vi "data beautifier.vi"(6 "Y-wave columns":u8[](array[numeric])=[4], 7 "X-wave column":u8, 8 "data cluster":cluster{"all rows":dbl[][]}[](array[cluster])=[{"all rows"=array3962x7[27734 elements]}, {"all rows"=array19075x7[133525 elements]}, {"all rows"=array4476x7[31332 elements]}], 9 "show files":T2(array[cluster])=[{"String"="sa_cryst,,_2nd.001", "Boolean"=TRUE, "begin"=0, "length"=3962, "y weight"=1.0}, {"String"="sa_cryst,,_2nd.002", "Boolean"=FALSE, "begin"=0, "length"=19075, "y weight"=1.0}, {"String"="sa_cryst,,_2nd.003", "Boolean"=TRUE, "begin"=0, "length"=4476, "y weight"=1.0}]) -> (0 "result data cluster":cluster{"all rows":dbl[][]}[](array[cluster]))   [LabVIEW 2019]
panel:
  in  "remove bad data pts":bool
  in  "remove duplicates":bool
  in  "cancel":bool
  in  "remove zero":bool
  out "XY Graph 2":T1(graph)
  in  "OK Button":bool
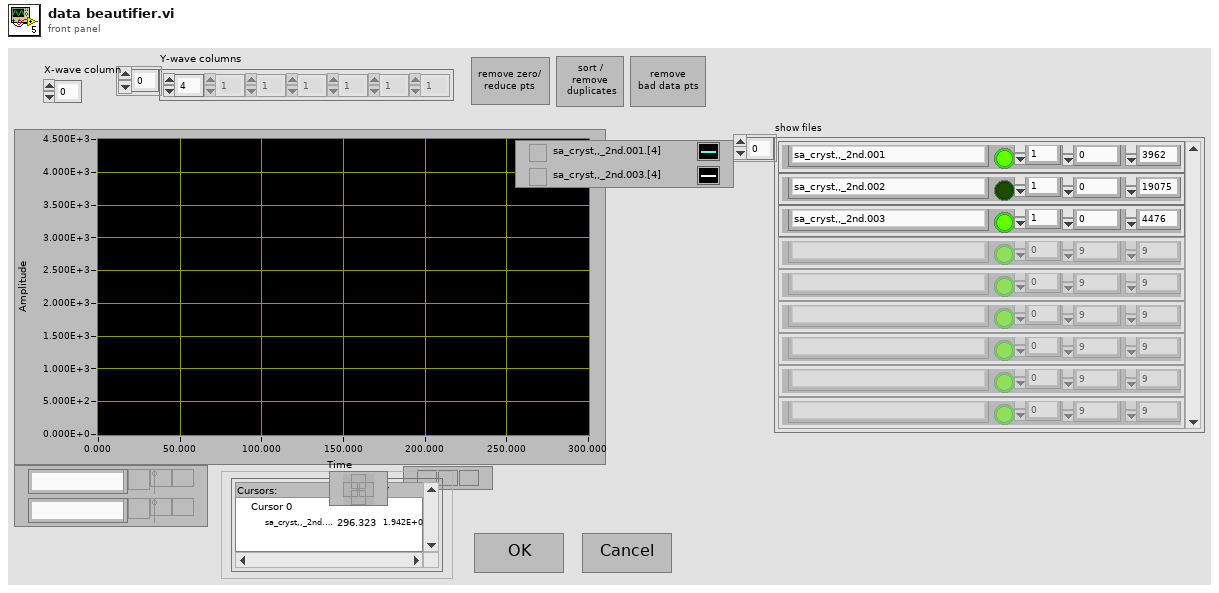
[diagram p1: front panel]
types:
  T1 = cluster{"indep array (x) out":dbl[], "dep array (y) out":dbl[]}[]
  T2 = cluster{"String":string, "Boolean":bool, "begin":u32, "length":u32, "y weight":dbl}[]
  T3 = cluster{"show files":cluster{"String":string, "Boolean":bool, "begin":u32, "length":u32, "y weight":dbl}[], "data cluster":cluster{"all rows":dbl[][]}[], "new dataset?":bool}
  T4 = cluster{"String":string, "Boolean":bool, "begin":u32, "end":u32, "Numeric":dbl}[]
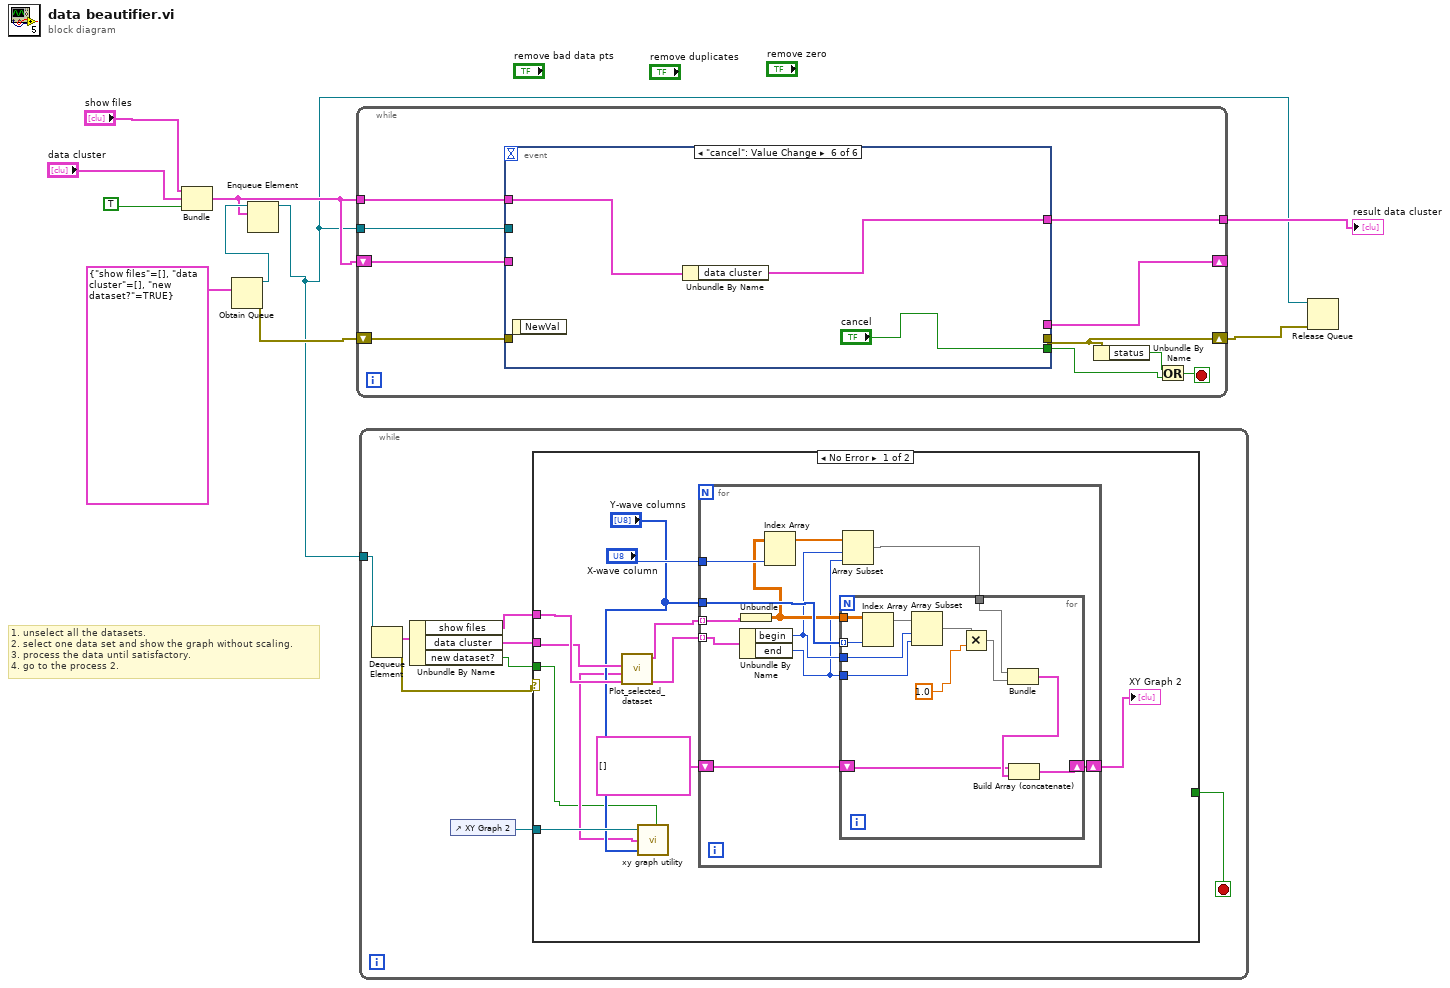
[diagram p0: block diagram]
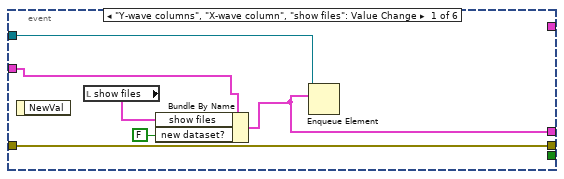
[diagram p2: hidden frame]
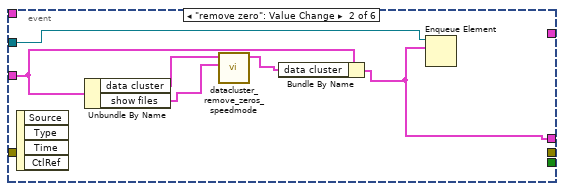
[diagram p3: hidden frame]
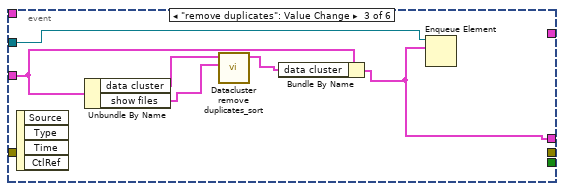
[diagram p4: hidden frame]
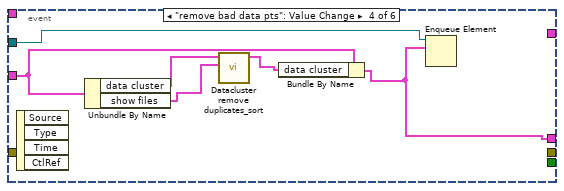
[diagram p5: hidden frame]
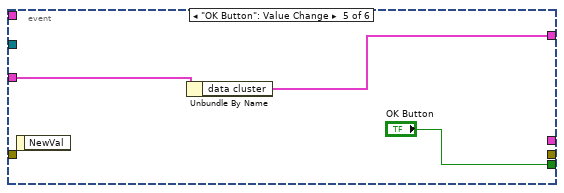
[diagram p6: hidden frame]
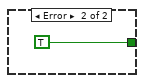
[diagram p7: hidden frame]
diagram:
  # "1. unselect all the datasets.\n2. select one data set and show the graph without scaling.\n3. process the data until satisfactory.\n4. go to the process 2."
  n1 = Bundle("show files"="show files", "data cluster"="data cluster", "new dataset?"=TRUE) -> (w3:T3)  [unwired: 1 in]
  n2 = Obtain Queue(element data type=T3 {"show files"=[], "data cluster"=[], "new dataset?"=TRUE}) -> (queue out=w4:refnum<queue>, error out=w9:errorcluster)  [unwired: 4 in, 1 out]
  n3 = Enqueue Element(queue=w4, element=w3) -> (queue out=w2:refnum<queue>)  [unwired: 2 in, 2 out]
  n4 = while {
    tunnel: w2 -> [w20]
    shift-right: [w19] -> _
    shift-left: w3 -> [w14]
    shift-right: [w13] -> w6
    shift-left: w9 -> [w18]
    tunnel: [w12] -> w5
    tunnel: w3 -> [w11]
    stop <- w15 stop-if-true
    n5 = event shown="[5] \"cancel\": Value Change" {
      selector: _ -> [_ _ _ _ _ _]
      dyn-events: _ -> [_ _ _ _ _ _]
      timeout: _ -> [_ _ _ _ _ _]
      tunnel: w20 -> [w26 w28 w34 w40 _ _]
      tunnel: [w23 w27 w33 w39 _ _] -> w19
      tunnel: w18 -> [w25 _ _ _ _ _]
      tunnel: [w25 _ _ _ _ _] -> w13
      tunnel: [_ _ _ _ "OK Button" "cancel"] -> w16
      tunnel: w14 -> [w22 w30 w36 w42 w46 _]
      tunnel: [_ _ _ _ w45 w50] -> w12
      tunnel: w11 -> [_ _ _ _ _ w48]
      event "Y-wave columns", "X-wave column", "show files": Value Change {
        n6 = event-data() -> ()  [unwired: 1 in, 1 out]
        n7 = local read "show files"() -> (w24:T2)
        n8 = Bundle By Name(cluster=w22, "show files"=w24, "new dataset?"=FALSE) -> (w23:T3)
        n9 = Enqueue Element(queue=w26, element=w23) -> ()  [unwired: 2 in, 3 out]
      }
      event "remove zero": Value Change {
        n10 = event-data() -> ()  [unwired: 1 in, 4 out]
        n11 = Unbundle By Name(w30) -> ("data cluster"=w31:cluster{"all rows":dbl[][]}[], "show files"=w32:T2)
        n12 = call "datacluster_remove_zeros_speedmode.vi"("Datasets to be processed"=w32, "data cluster"=w31) -> ("data cluster out"=w29:cluster{"all rows":dbl[][]}[])  [unwired: 9 in]
        n13 = Bundle By Name(cluster=w30, "data cluster"=w29) -> (w27:T3)
        n14 = Enqueue Element(queue=w28, element=w27) -> ()  [unwired: 2 in, 3 out]
      }
      event "remove duplicates": Value Change {
        n15 = event-data() -> ()  [unwired: 1 in, 4 out]
        n16 = Unbundle By Name(w36) -> ("data cluster"=w37:cluster{"all rows":dbl[][]}[], "show files"=w38:T2)
        n17 = call "Datacluster remove duplicates_sort.vi"("Datasets to be processed"=w38, "data cluster"=w37) -> ("data cluster out"=w35:cluster{"all rows":dbl[][]}[])  [unwired: 9 in]
        n18 = Bundle By Name(cluster=w36, "data cluster"=w35) -> (w33:T3)
        n19 = Enqueue Element(queue=w34, element=w33) -> ()  [unwired: 2 in, 3 out]
      }
      event "remove bad data pts": Value Change {
        n20 = event-data() -> ()  [unwired: 1 in, 4 out]
        n21 = Unbundle By Name(w42) -> ("data cluster"=w43:cluster{"all rows":dbl[][]}[], "show files"=w44:T2)
        n22 = call "Datacluster remove duplicates_sort.vi"("Datasets to be processed"=w44, "data cluster"=w43) -> ("data cluster out"=w41:cluster{"all rows":dbl[][]}[])  [unwired: 9 in]
        n23 = Bundle By Name(cluster=w42, "data cluster"=w41) -> (w39:T3)
        n24 = Enqueue Element(queue=w40, element=w39) -> ()  [unwired: 2 in, 3 out]
      }
      event "OK Button": Value Change {
        n25 = event-data() -> ()  [unwired: 1 in, 1 out]
        n26 = Unbundle By Name(w46) -> ("data cluster"=w45:cluster{"all rows":dbl[][]}[])
      }
      event "cancel": Value Change {
        n27 = event-data() -> ()  [unwired: 1 in, 1 out]
        n28 = Unbundle By Name(w48) -> ("data cluster"=w50:cluster{"all rows":dbl[][]}[])
      }
    }
    n29 = Unbundle By Name(w13) -> ("status"=w17:bool)
    n30 = Or(x=w17, y=w16) -> (x .or. y?=w15:bool)
  }
  "result data cluster" <- w5
  n31 = while {
    tunnel: w2 -> [w58]
    stop <- w53 stop-if-true
    n32 = Dequeue Element(queue=w58) -> (element=w57:T3, error out=w54:errorcluster)  [unwired: 2 in, 2 out]
    n33 = Unbundle By Name(w57) -> ("show files"=w55:T2, "data cluster"=w56:cluster{"all rows":dbl[][]}[], "new dataset?"=w51:bool)
    n34 = control-ref of="XY Graph 2"() -> (w52:refnum<vi>)
    n35 = case shown="No Error" w54 {
      tunnel: w56 -> [w64 _]
      tunnel: w55 -> [w65 _]
      tunnel: [_ TRUE] -> w53
      tunnel: w52 -> [w62 _]
      tunnel: w51 -> [w59 _]
      frame No Error {
        n36 = call "Plot_selected_dataset.vi"("input xy data arrays"=w64, "file names and switch"=w65) -> ("show files out"=w60:T4, "selected xy data arrays"=w63:cluster{"all rows":dbl[][]}[], "selected showfiles"=w66:T4)  [unwired: 1 in, 4 out]
        n37 = call "xy graph utility.vi"("redraw?"=w59, "y-wave columns"="Y-wave columns", "show files"=w60, "XYGraph Refnum"=w62) -> ()  [unwired: 1 in]
        n38 = for {
          tunnel: "Y-wave columns" -> [w80]
          tunnel: "X-wave column" -> [w79]
          tunnel: w63 -> [w72] mode=indexing
          tunnel: w66 -> [w71] mode=indexing
          shift-right: [w73] -> w68
          shift-left: cluster{dbl[], dbl[]}[] [] -> [w70]
          n39 = Unbundle By Name(w71) -> ("begin"=w76:u32, "end"=w75:u32)
          n40 = Unbundle(w72) -> ("all rows"=w78:dbl[][])
          n41 = Index Array(array=w78, index (col)=w79) -> (element=w77:dbl[])  [unwired: 1 in]
          n42 = Array Subset(array=w77, index=w76, length=w75) -> (w74:dbl[])
          n43 = for {
            tunnel: w78 -> [w92]
            tunnel: w80 -> [w91] mode=indexing
            tunnel: w76 -> [w89]
            tunnel: w75 -> [w88]
            tunnel: w74 -> [w83]
            shift-right: [w84] -> w73
            shift-left: w70 -> [w85]
            n44 = Index Array(array=w92, index (col)=w91) -> (element=w90:dbl[])  [unwired: 1 in]
            n45 = Array Subset(array=w90, index=w89, length=w88) -> (w87:dbl[])
            n46 = Multiply(x=w87, y=1.0) -> (x*y=w82:dbl[])
            n47 = Bundle(w83, w82) -> (w86:cluster{dbl[], dbl[]})  [unwired: 1 out]
            n48 = Build Array (concatenate)(w85, w86) -> (w84:cluster{dbl[], dbl[]}[])
          }
        }
        "XY Graph 2" <- w68
      }
      frame Error {
      }
    }
  }
  n49 = Release Queue(queue=w2, error in (no error)=w6) -> ()  [unwired: 1 in, 3 out]
